vi "Inject_Av_Advection_Vel.vi"() -> (0 "New Values In":string[][](array[string])=[["Test data5"]], 1 "New Chs In":string[](array[string])=["30-10-03:New:Channel new5"])   [LabVIEW 2011]
uses:
  Results_plotter_Global.vi
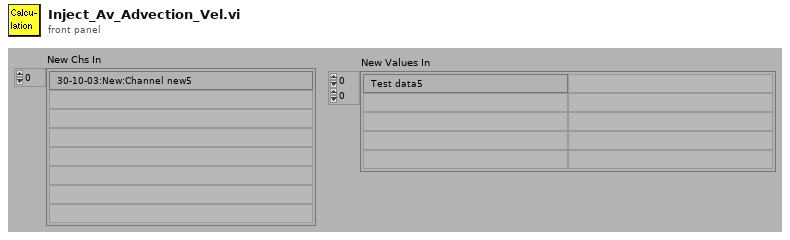
[diagram p1: front panel]
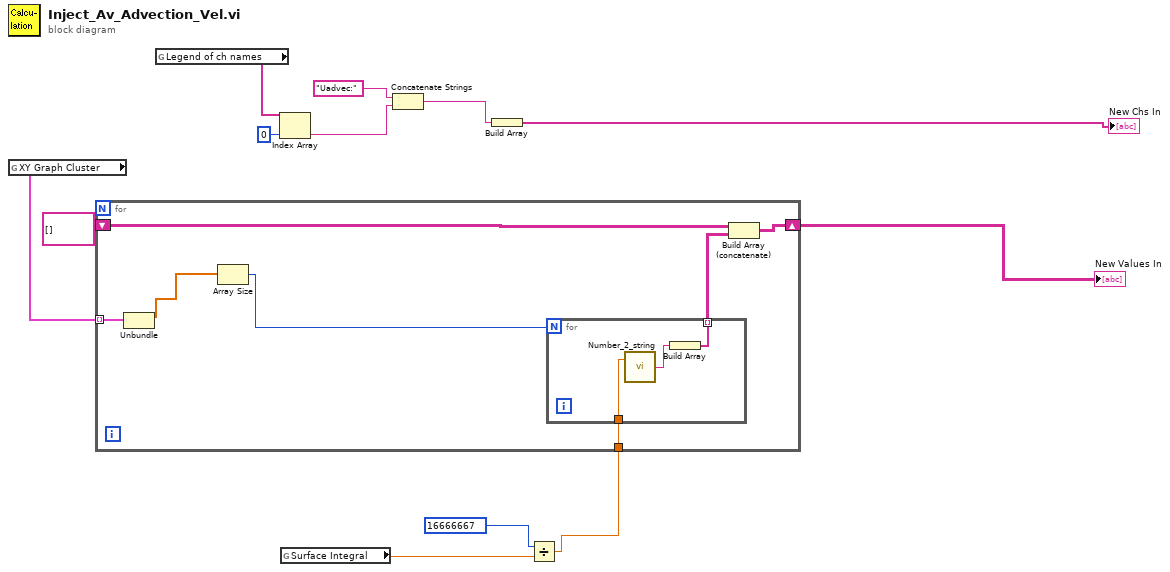
[diagram p0: block diagram]
diagram:
  n1 = global read "Results_plotter_Global.vi" "XY Graph Cluster"() -> (w12:cluster{dbl[], dbl[]}[])
  n2 = global read "Results_plotter_Global.vi" "Legend of ch names"() -> (w10:string[])
  n3 = Index Array(array=w10, index=0) -> (element=w6:string)
  n4 = global read "Results_plotter_Global.vi" "Surface Integral"() -> (w2:dbl)
  n5 = Concatenate Strings("Uadvec:" ("string"), w6) -> (w8:string)
  n6 = Build Array(w8) -> (→"New Chs In":string[])
  n7 = Divide(x=16666667, y=w2) -> (x/y=w1:dbl)
  n8 = for {
    tunnel: w12 -> [w19] mode=indexing
    shift-right: [w16] -> w4
    shift-left: string[][] [] -> [w18]
    tunnel: w1 -> [w13]
    n9 = Unbundle(w19) -> (w15:dbl[])  [unwired: 1 out]
    n10 = Array Size(array=w15) -> (size(s)=w14:i32)
    n11 = for {
      N: w14 -> [_]
      tunnel: [w21] -> w17 mode=indexing
      tunnel: w13 -> [w20]
      n12 = call "Number_2_string.vi"("number"=w20) -> ("String"=w22:string)  [unwired: 1 in]
      n13 = Build Array(w22) -> (w21:string[])
    }
    n14 = Build Array (concatenate)(w18, w17) -> (w16:string[][])
  }
  "New Values In" <- w4
